vi "FilePath.vi"() -> ()   [LabVIEW 2019]
panel:
  in  "Path":path
  # "Path to CommandTemplates folder"
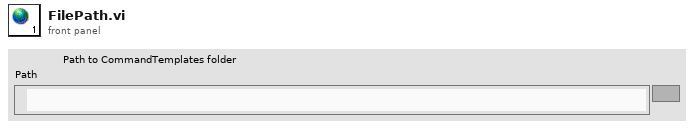
[diagram p1: front panel]
diagram:
